vi "PmSetExternalTrigger.vi"(8 "error in (no error)":errorcluster, 10 "Trigger Setting":T1(ring), 11 "reference":refnum<k24>) -> (0 "error out":errorcluster, 3 "reference out":refnum<k24>)   [LabVIEW 2022 SP3, in "Photometrics Camera.lvlib"]
uses:
  Photometrics Camera.lvlib
  C:/FlashGordon/Development/dll/PVCamNET.dll
  dll/PVCamNET.dll
panel:
  out "Trigger":string
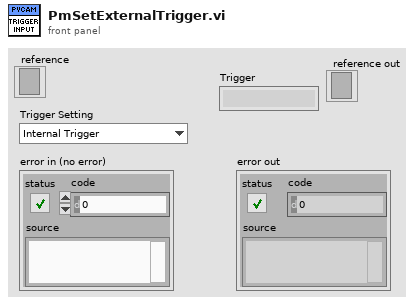
[diagram p1: front panel]
types:
  T1 = enum32{"Internal Trigger", "Edge Trigger", "Trigger First", "Level Trigger", "Level Trigger Overlap", "Software Trigger Edges", "Software Trigger First"}
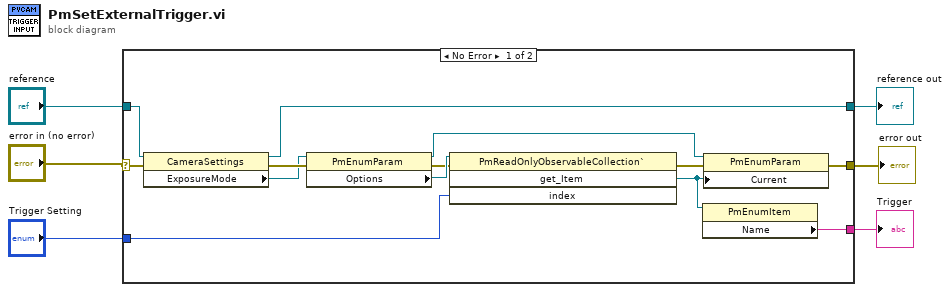
[diagram p0: block diagram]
diagram:
  n1 = case shown="No Error" "error in (no error)" {
    selector: "error in (no error)" -> [w15 w21]
    tunnel: "reference" -> [w17 w20]
    tunnel: [w14 w21] -> w5
    tunnel: [w16 w20] -> w4
    tunnel: "Trigger Setting" -> [w11 _]
    tunnel: [w7 _] -> w1
    frame No Error {
      n2 = property class="CameraSettings"(reference=w17, error in=w15) -> (reference out=w16:refnum<k24>, error out=w19:errorcluster, "ExposureMode"=w18:refnum<k24>)
      n3 = property class="PmEnumParam"(reference=w18, error in=w19) -> (reference out=w12:refnum<k24>, error out=w10:errorcluster, "Options"=w13:refnum<k24>)
      n4 = invoke class="PmReadOnlyObservableCollection`" method="get_Item"(reference=w13, error in=w10, "index"=w11) -> (error out=w9:errorcluster, "get_Item"=w8:refnum<k24>)  [unwired: 1 in, 2 out]
      n5 = property class="PmEnumItem"(reference=w8) -> ("Name"=w7:string)  [unwired: 1 in, 2 out]
      n6 = property class="PmEnumParam"(reference=w12, error in=w9, "Current"=w8) -> (error out=w14:errorcluster)  [unwired: 1 out]
    }
    frame Error {
    }
  }
  "error out" <- w5
  "reference out" <- w4
  "Trigger" <- w1
